vi "Fire_alarm_A1.vi"() -> ()   [LabVIEW 2020]
panel:
  out "Flame":dbl(slide) scale=0.0..1.0
  in  "VISA resource name":refnum<visa-resource-name>
  out "Smoke Chart":dbl(graph)
  out "Flame":bool
  out "Smoke":bool
  out "Fire Indicator":bool
  out "Flame Chart":dbl(graph)
  out "Smoke 4":dbl(slide) scale=0.0..1.0
  in  "Table Control":string[][](table)
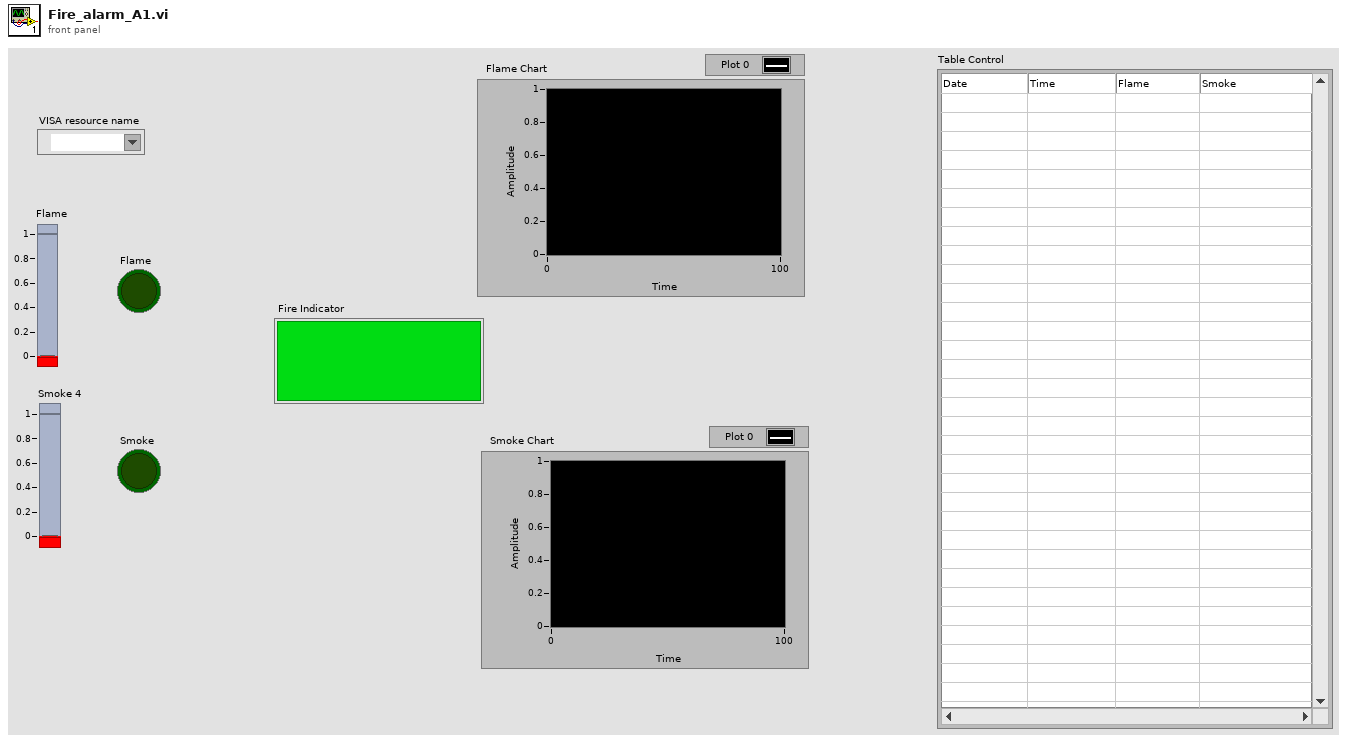
[diagram p1: front panel]
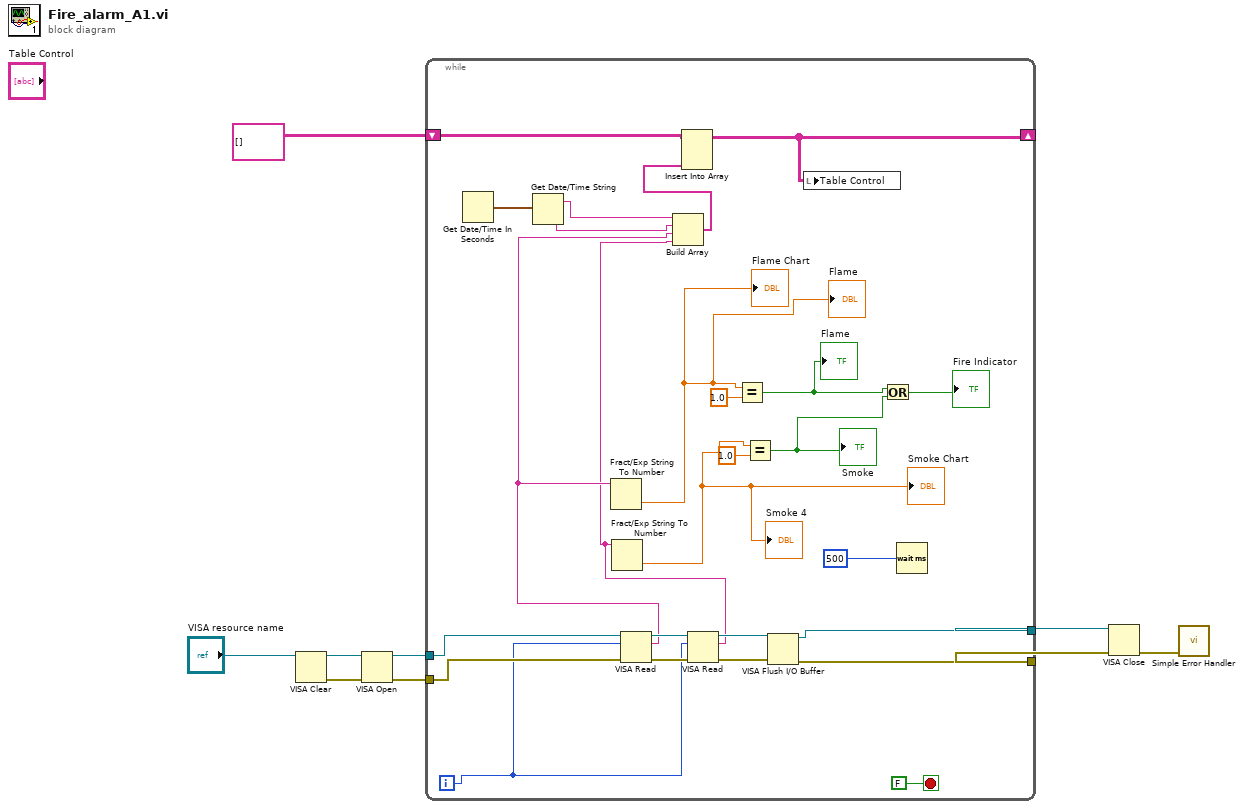
[diagram p0: block diagram]
diagram:
  n1 = VISA Clear(VISA resource name="VISA resource name") -> (VISA resource name out=w9:refnum<visa-resource-name>, error out=w8:errorcluster)  [unwired: 1 in]
  n2 = VISA Open(error in (no error)=w8, VISA resource name=w9) -> (VISA resource name=w7:refnum<visa-resource-name>, error out=w6:errorcluster)  [unwired: 3 in]
  n3 = while {
    tunnel: w7 -> [w35]
    tunnel: w6 -> [w34]
    tunnel: [w29] -> w5
    tunnel: [w28] -> w4
    shift-right: [w24] -> _
    shift-left: string[][] [] -> [w25]
    i -> [w27]
    stop <- FALSE stop-if-true
    n4 = Get Date/Time In Seconds() -> (seconds since 1Jan1904=w23:timestamp)
    n5 = Get Date/Time String(seconds (now)=w23) -> (date string=w22:string, time string=w21:string)  [unwired: 2 in]
    n6 = VISA Read(VISA resource name=w35, byte count=w27, error in (no error)=w34) -> (VISA resource name out=w33:refnum<visa-resource-name>, read buffer=w20:string, error out=w32:errorcluster)  [unwired: 1 out]
    n7 = Fract/Exp String To Number(string=w20) -> (number=w13:dbl)  [unwired: 3 in, 1 out]
    "Flame Chart" <- w13
    "Flame" <- w13
    n8 = VISA Read(VISA resource name=w33, byte count=w27, error in (no error)=w32) -> (VISA resource name out=w31:refnum<visa-resource-name>, read buffer=w19:string, error out=w30:errorcluster)  [unwired: 1 out]
    n9 = Fract/Exp String To Number(string=w19) -> (number=w14:dbl)  [unwired: 3 in, 1 out]
    "Smoke Chart" <- w14
    "Smoke 4" <- w14
    n10 = Build Array(w22, w21, w20, w19) -> (w18:string[])
    n11 = Insert Into Array(array=w25, new element=w18) -> (w24:string[][])  [unwired: 2 in]
    n12 = Equal?(x=w13, y=1.0) -> (x = y?=w12:bool)
    "Flame" <- w12
    n13 = Equal?(x=w14, y=1.0) -> (x = y?=w11:bool)
    "Smoke" <- w11
    n14 = VISA Flush I/O Buffer(VISA resource name=w31, error in (no error)=w30) -> (VISA resource name out=w29:refnum<visa-resource-name>, error out=w28:errorcluster)  [unwired: 1 in]
    n15 = local write "Table Control"(w24) -> ()
    n16 = Or(x=w12, y=w11) -> (x .or. y?=→"Fire Indicator":bool)
    n17 = Wait (ms)(milliseconds to wait=u32 500) -> ()  [unwired: 1 out]
  }
  n18 = VISA Close(VISA resource name=w5, error in (no error)=w4) -> (error out=w3:errorcluster)
  n19 = call <vilib>:"Simple Error Handler.vi"("error in (no error)"=w3) -> ()  [unwired: 4 in, 5 out]
